vi "Initialize_FP_Input Ranges CH1.vi"(8 "error in (no error)":errorcluster) -> (0 "error out":errorcluster)   [LabVIEW 2019]
panel:
  # "--- Inputs ---"
  # "--- Outputs ---"
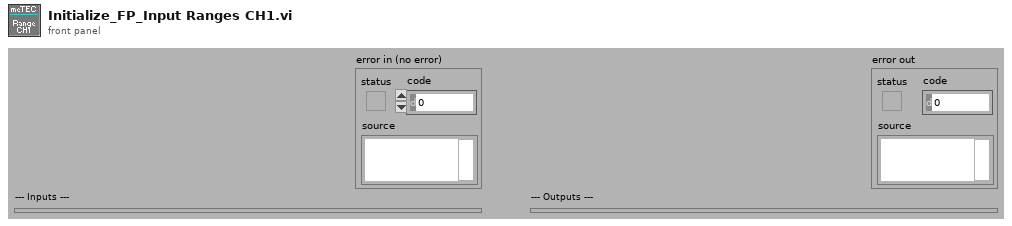
[diagram p1: front panel]
types:
  T1 = typedef "FGV_TE Controller.ctl" = cluster{"SVs":cluster{"Unused":dbl}, "PVs":cluster{"FW & HW Versions":cluster{"Device Type [I32]":i32, "Device Type [String]":string, "Firmware Version [I32]":i32, "Firmware Version [String]":string, "Hardware Version [I32]":i32, "Hardware Version [String]":string, "Serial No.":i32}, "TEC Configuration":T2, "Object Target Temperature Source_CH1":u8, "Object Target Temperature Source_CH2":u8}, "Front Panel References":T3}
  T2 = typedef "meTEC_Configuration.ctl" = cluster{"VISA resource name":refnum<visa-resource-name>, "Device Address":u16}
  T3 = typedef "FGV_Front Panel References.ctl" = cluster{"Main Loop Queue":refnum<queue>, "meTEC_Device Type":refnum<vi>, "meTEC_Serial No.":refnum<vi>, "meTEC_Hardware Version":refnum<vi>, "meTEC_Firmware Version":refnum<vi>, "meTEC_CH1_Object Target Temperature (ID 3000 / 50012) [°C]":refnum<vi>, "meTEC_CH1_Live Set Current (ID 50001) [A]":refnum<vi>, "meTEC_CH1_Live Set Voltage (ID 50002) [V]":refnum<vi>, "meTEC_CH1_Live Enable (ID 50000)":refnum<vi>, "meTEC_CH1_Input Selection (ID 2000)":refnum<vi>, "meTEC_CH1_Object Target Temp. Source Sel. (ID 50011)":refnum<vi>, "meTEC_CH2_Object Target Temperature (ID 3000 / 50012) [°C]":refnum<vi>, "meTEC_CH2_Live Set Current (ID 50001) [A]":refnum<vi>, "meTEC_CH2_Live Set Voltage (ID 50002) [V]":refnum<vi>, "meTEC_CH2_Live Enable (ID 50000)":refnum<vi>, "meTEC_CH2_Input Selection (ID 2000)":refnum<vi>, "meTEC_CH2_Object Target Temp. Source Sel. (ID 50011)":refnum<vi>, "meTEC_CH2_Object Temperature [°C]":refnum<vi>, "meTEC_CH2_Sink Temperature [°C]":refnum<vi>, "meTEC_CH2_Act. Output Current [A]":refnum<vi>, "meTEC_CH2_Act. Output Voltage [V]":refnum<vi>, "meTEC_CH2_Temperature Stability":refnum<vi>, "Monitor Chart_CH2":refnum<vi>, "meTEC_Initialize Device":refnum<vi>}
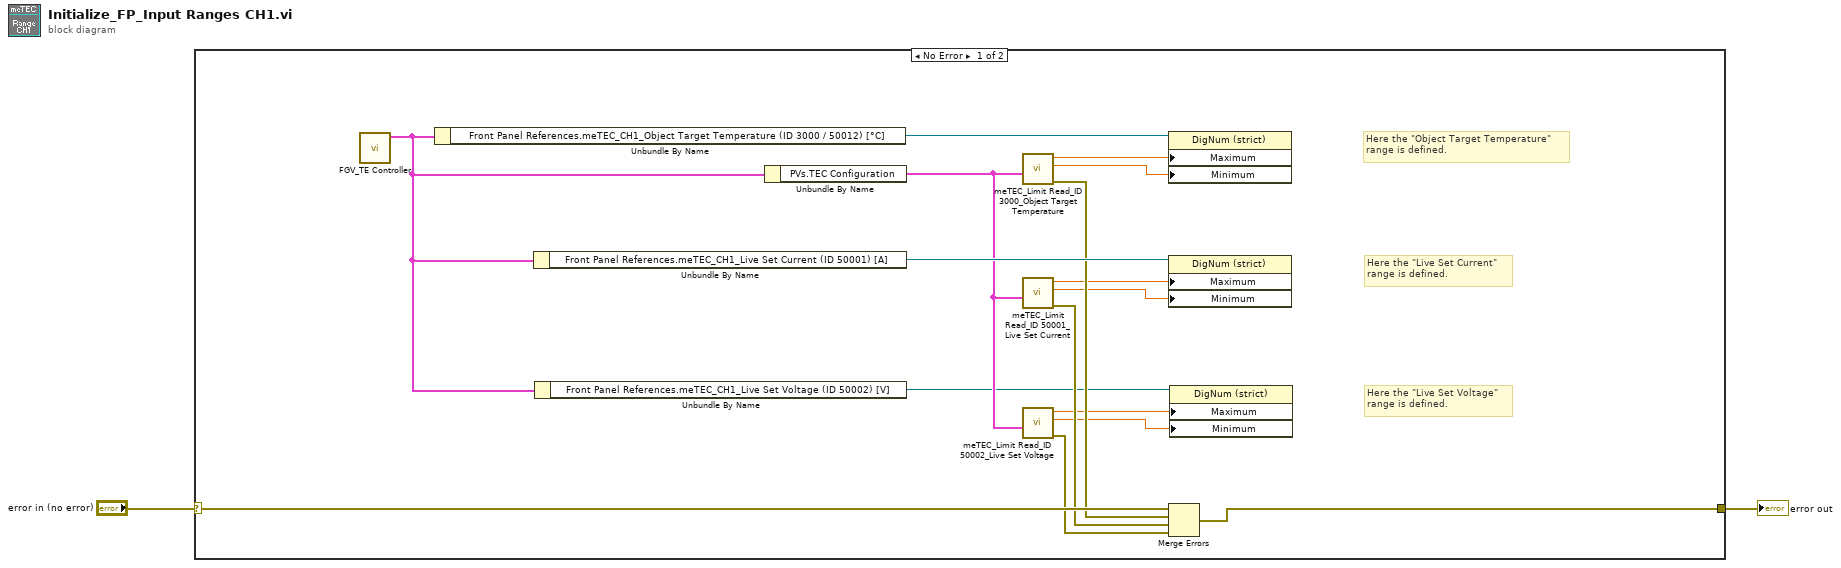
[diagram p0: block diagram]
diagram:
  n1 = case shown="No Error" "error in (no error)" {
    selector: "error in (no error)" -> [w18 w19]
    tunnel: [w6 w19] -> w2
    frame No Error {
      # "Here the \"Object Target Temperature\" \nrange is defined."
      # "Here the \"Live Set Voltage\" \nrange is defined."
      # "Here the \"Live Set Current\" \nrange is defined."
      n2 = call "FGV_TE Controller.vi"() -> ("FGV_TEC_OUT"=w16:T1)  [unwired: 10 in, 1 out]
      n3 = Unbundle By Name(w16) -> ("Front Panel References.meTEC_CH1_Object Target Temperature (ID 3000 / 50012) [°C]"=w17:refnum<vi>)
      n4 = Unbundle By Name(w16) -> ("Front Panel References.meTEC_CH1_Live Set Current (ID 50001) [A]"=w15:refnum<vi>)
      n5 = Unbundle By Name(w16) -> ("Front Panel References.meTEC_CH1_Live Set Voltage (ID 50002) [V]"=w9:refnum<vi>)
      n6 = Unbundle By Name(w16) -> ("PVs.TEC Configuration"=w10:T2)
      n7 = call "meTEC_Limit Read_ID 3000_Object Target Temperature.vi"("TEC Configuration_IN"=w10) -> ("error out"=w13:errorcluster, "Temperature Input Range_Min. [°C]"=w5:dbl, "Temperature Input Range_Max. [°C]"=w14:dbl)  [unwired: 7 in, 1 out]
      n8 = call "meTEC_Limit Read_ID 50001_Live Set Current.vi"("TEC Configuration_IN"=w10) -> ("error out"=w12:errorcluster, "Current Input Range_Min. [A]"=w4:dbl, "Current Input Range_Max. [A]"=w11:dbl)  [unwired: 7 in, 1 out]
      n9 = call "meTEC_Limit Read_ID 50002_Live Set Voltage.vi"("TEC Configuration_IN"=w10) -> ("error out"=w7:errorcluster, "Voltage Input Range_Min. [V]"=w3:dbl, "Voltage Input Range_Max. [V]"=w8:dbl)  [unwired: 7 in, 1 out]
      n10 = property class="DigNum (strict)"(reference=w17, "Maximum"=w14, "Minimum"=w5) -> ()  [unwired: 1 in, 2 out]
      n11 = property class="DigNum (strict)"(reference=w15, "Maximum"=w11, "Minimum"=w4) -> ()  [unwired: 1 in, 2 out]
      n12 = Merge Errors(w18, w13, w12, w7) -> (w6:errorcluster)
      n13 = property class="DigNum (strict)"(reference=w9, "Maximum"=w8, "Minimum"=w3) -> ()  [unwired: 1 in, 2 out]
    }
    frame Error {
    }
  }
  "error out" <- w2
